vi "X_Y_Relation.vi"() -> ()   [LabVIEW 2025]
panel:
  out "X in relation to Y":string
  in  "Y":dbl
  in  "X":dbl
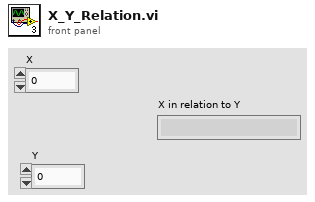
[diagram p1: front panel]
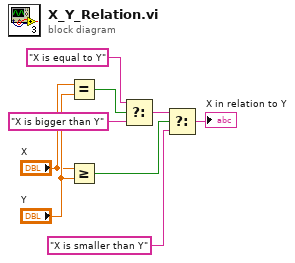
[diagram p0: block diagram]
diagram:
  n1 = Equal?(x="X", y="Y") -> (x = y?=w9:bool)
  n2 = Greater Or Equal?(x="X", y="Y") -> (x >= y?=w5:bool)
  n3 = Select(t="X is equal to Y", s=w9, f="X is bigger than Y") -> (s? t:f=w2:string)
  n4 = Select(t=w2, s=w5, f="X is smaller than Y") -> (s? t:f=→"X in relation to Y":string)
